vi "Max_Error_Calculator.vi"(10 "数值":sgl format="%#.2g", 11 "数组":sgl[](array[numeric]) format="%#.2g") -> (2 "dev":sgl format="%#.2g", 3 "inaccc":sgl format="%#.2g")   [LabVIEW 2019]
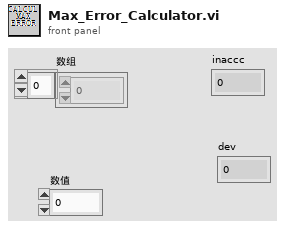
[diagram p1: front panel]
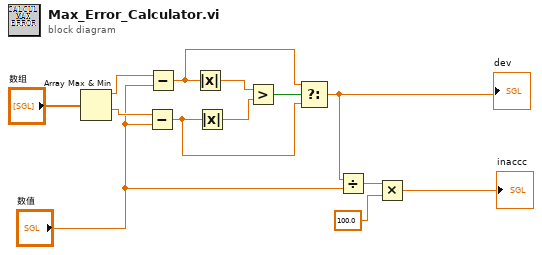
[diagram p0: block diagram]
diagram:
  n1 = Array Max & Min(array="数组") -> (max value=w12:sgl, min value=w11:sgl)  [unwired: 2 out]
  n2 = Subtract(x=w11, y="数值") -> (x-y=w2:sgl)
  n3 = Subtract(x=w12, y="数值") -> (x-y=w1:sgl)
  n4 = Absolute Value(x=w1) -> (abs(x)=w9:sgl)
  n5 = Absolute Value(x=w2) -> (abs(x)=w3:sgl)
  n6 = Greater?(x=w9, y=w3) -> (0:w10:bool)
  n7 = Select(t=w1, s=w10, f=w2) -> (s? t:f=w8:sgl)
  "dev" <- w8
  n8 = Divide(x=w8, y="数值") -> (x/y=w6:sgl)
  n9 = Multiply(x=w6, y=sgl 100.0) -> (x*y=→"inaccc":sgl)
